vi "Write Next Column.vi"(8 "error in (no error)":errorcluster, 10 "Next Column":i32, 11 "SQL Statement in":refnum<class "SQL Statement.lvclass">) -> (0 "error out":errorcluster, 3 "SQL Statement out":refnum<class "SQL Statement.lvclass">)   [LabVIEW 2023, in "SQLite.lvlib" / "SQL Statement.lvclass"]
doc: "Sets the index of the next column to get. Note that this index self-increments with each column \"gotten\", so this function is not necessarily needed."
uses:
  SQL Statement.lvclass
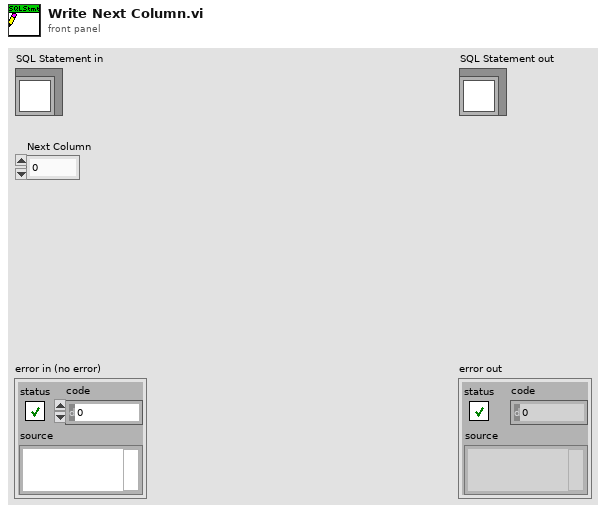
[diagram p1: front panel]
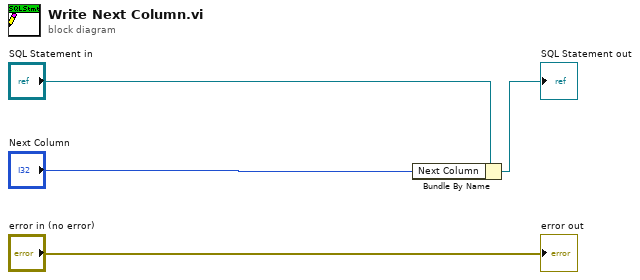
[diagram p0: block diagram]
diagram:
  n1 = Bundle By Name(cluster="SQL Statement in", "Next Column"="Next Column") -> (→"SQL Statement out":refnum<class "SQL Statement.lvclass">)
  "error out" <- "error in (no error)"
